vi "get key switch state.vi"(8 "error in (no error)":errorcluster, 11 "Cobolt in":refnum<class "Cobolt.lvclass">) -> (0 "error out":errorcluster, 3 "Cobolt out":refnum<class "Cobolt.lvclass">)   [LabVIEW 2012, in "Cobolt.lvclass"]
uses:
  Cobolt.lvclass
  CoboltLaserDrivers_Public_LV2012/CoboltLaser_Controls/ExpectedResponseType.ctl
  Cobolt.lvclass/Cobolt.ctl
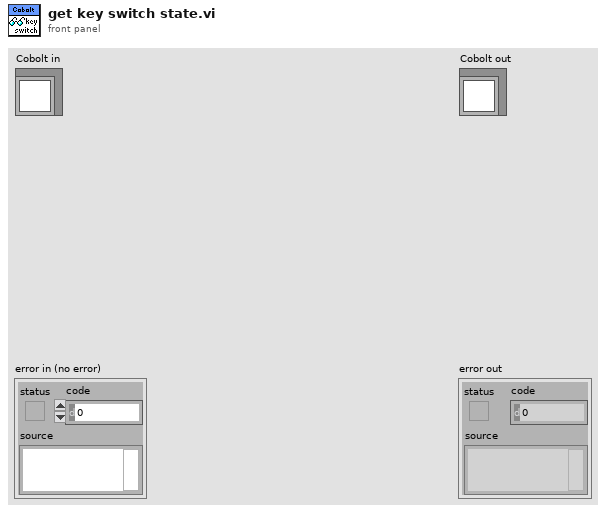
[diagram p1: front panel]
types:
  T1 = typedef "Cobolt.lvclass/ExpectedResponseType.ctl" = u16
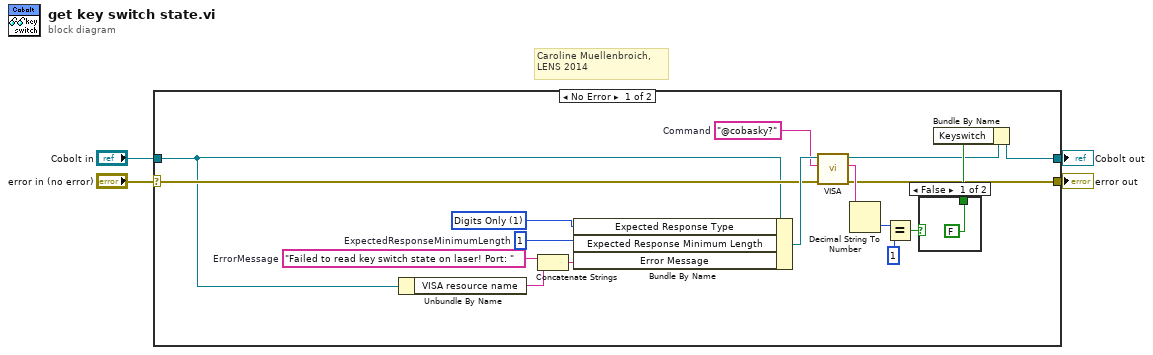
[diagram p0: block diagram]
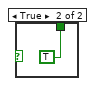
[diagram p2: hidden frame]
diagram:
  # "Caroline Muellenbroich, \nLENS 2014"
  n1 = case shown="No Error" "error in (no error)" {
    selector: "error in (no error)" -> [w8 w25]
    tunnel: [w7 w25] -> w3
    tunnel: [w5 w24] -> w1
    tunnel: "Cobolt in" -> [w6 w24]
    frame No Error {
      w16 = T1 1 items=["Any", "Digits Only", "Non-Digits Only"] ("ExpectedResponseType")
      w12 = 1  # ExpectedResponseMinimumLength
      w14 = "Failed to read key switch state on laser! Port: "  # ErrorMessage
      w10 = "@cobasky?"  # Command
      n2 = Unbundle By Name(w6) -> ("VISA resource name"=w13:string)
      n3 = Concatenate Strings(w14, w13) -> (w15:string)
      n4 = Bundle By Name(cluster=w6, "Expected Response Type"=w16, "Expected Response Minimum Length"=w12, "Error Message"=w15) -> (w11:refnum<class "Cobolt.lvclass">)
      n5 = call-dynamic "VISA.vi"("error in (no error)"=w8, "string to write"=w10, "Cobolt in"=w11) -> ("error out"=w7:errorcluster, "buffer out"=w19:string, "Cobolt out"=w9:refnum<class "Cobolt.lvclass">)  [unwired: 6 in]
      n6 = Decimal String To Number(string=w19) -> (number=w18:i32)  [unwired: 2 in, 1 out]
      n7 = Equal?(x=w18, y=1) -> (x = y?=w20:bool)
      n8 = case shown="False" w20 {
        tunnel: [FALSE TRUE] -> w21
        frame False {
        }
        frame True {
        }
      }
      n9 = Bundle By Name(cluster=w9, "Keyswitch"=w21) -> (w5:refnum<class "Cobolt.lvclass">)
    }
    frame Error {
    }
  }
  "error out" <- w3
  "Cobolt out" <- w1
